vi "Pickering 4 wire PPMS Puck.vi"(8 "error in (no error)":errorcluster, 10 "Channel Cluster":T1={"26"=["NC"], "27"=["NC"], "28"=["NC", "NC"], "1"=["NC"], "2"=["NC"], "3"=["NC"], "4"=["NC"], "5"=["NC"], "24"=["NC"], "25"=["NC"], "6"=["NC"]}) -> (0 "error out":errorcluster)   [LabVIEW 2016, in "pickering.lvclass"]
uses:
  pickering.lvclass
panel:
  in  "Initialize":bool
  in  "Pickering status":path=path "C:/LabView/PPMS basic VIs/Switch Status.txt"
  in  "Disconnect all?":bool
  in  "IVI Option String":string="Simulate=0,RangeCheck=1,QueryInstrStatus=0,Cache=1,DriverSetup=Model:40-726-511-M;"
  in  "VISA Resource Name":string="PXI9::13::INSTR"
  # "2"
  # "6"
  # "25"
  # "24"
  # "5"
  # "4"
  # "3"
  # "26"
  # "27"
  # "28"
  # "1"
  # "4 wire              measurements\nFeature:\n1, Multiple connections\n2, Make before break\n3, First run resets device\n\nNotes:\nLock-in 1: I+/I- -->AO0/AI0, board 0\n\nLock-in 3: V+/V-  --> AI0, board 1.  \n  V+/V- conencted to y3 and y4. OSC output should set the same as Lock-in 1\n\nLock-in 2: I2+/I2- -->AO1/AI1, board 0\n\nLock-in 4: V2+/V2- -> y7/y8"
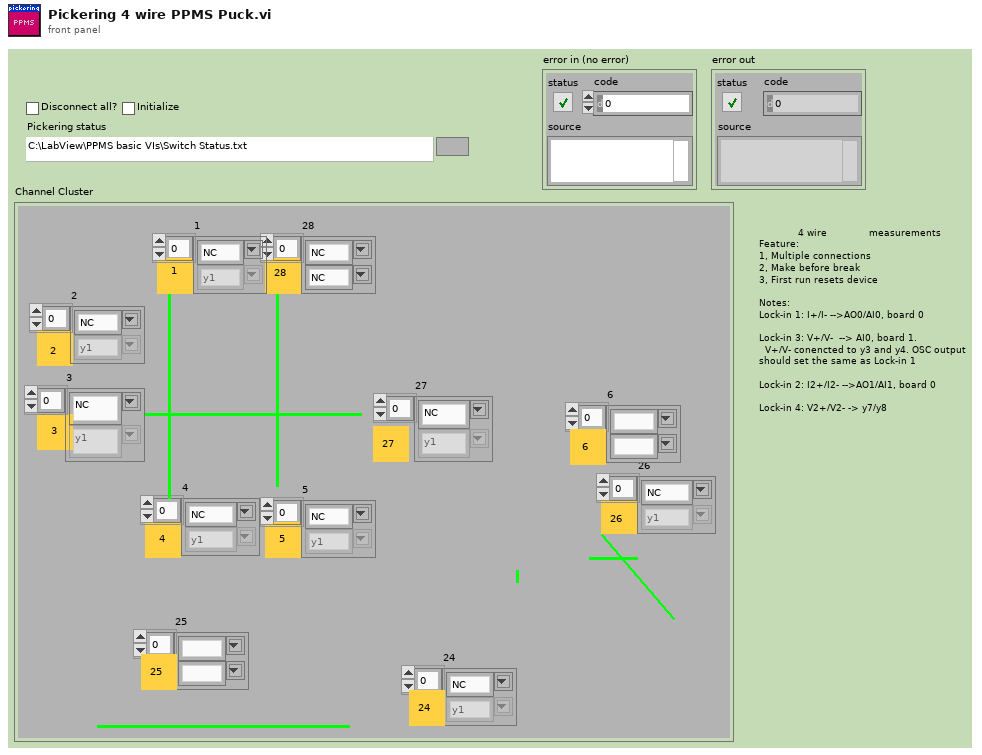
[diagram p1: front panel]
types:
  T1 = cluster{"26":string[], "27":string[], "28":string[], "1":string[], "2":string[], "3":string[], "4":string[], "5":string[], "24":string[], "25":string[], "6":string[]}
  T2 = cluster{"Initialize":bool, "Disconnect all?":bool, "Discharge X channels?":bool, "Discharge Y Channels?":bool}
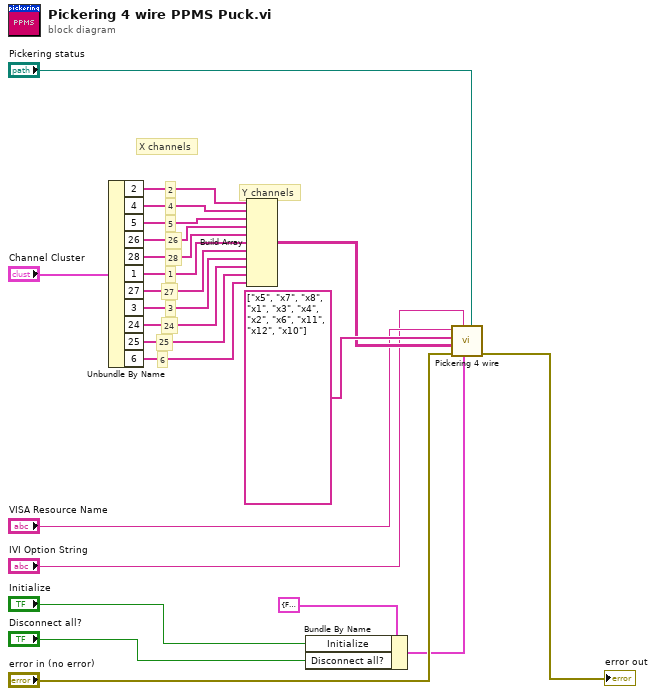
[diagram p0: block diagram]
diagram:
  # "6"
  # "25"
  # "X channels"
  # "Y channels"
  # "24"
  # "3"
  # "27"
  # "1"
  # "28"
  # "26"
  # "5"
  # "4"
  # "2"
  n1 = Unbundle By Name("Channel Cluster") -> ("2"=w11:string[], "4"=w10:string[], "5"=w9:string[], "26"=w8:string[], "28"=w7:string[], "1"=w6:string[], "27"=w5:string[], "3"=w4:string[], "24"=w3:string[], "25"=w2:string[], "6"=w1:string[])
  n2 = Build Array(w11, w10, w9, w8, w7, w6, w5, w4, w3, w2, w1) -> (w22:string[][])
  n3 = Bundle By Name(cluster=T2 {"Initialize"=FALSE, "Disconnect all?"=FALSE, "Discharge X channels?"=TRUE, "Discharge Y Channels?"=TRUE} ("configuration"), "Initialize"="Initialize", "Disconnect all?"="Disconnect all?") -> (w13:T2)
  n4 = call "Pickering 4 wire.vi"("Pickering status"="Pickering status", "configuration"=w13, "IVI Option String"="IVI Option String", "error in (no error)"="error in (no error)", "Y Channels"=w22, "X Channels"=string[] ["x5", "x7", "x8", "x1", "x3", "x4", "x2", "x6", "x11", "x12", "x10"], "VISA Resource Name"="VISA Resource Name") -> ("error out"=→"error out":errorcluster)  [unwired: 3 in, 1 out]
